vi "set active buffer.vi"(8 "error in (no error)":errorcluster, 11 "Thorcam in":refnum<class "Thorcam.lvclass">) -> (0 "error out":errorcluster, 3 "Thorcam out":refnum<class "Thorcam.lvclass">)   [LabVIEW 2012, in "Thorcam.lvclass"]
uses:
  Thorcam.lvclass
  Thorcam.lvclass/Thorcam.ctl
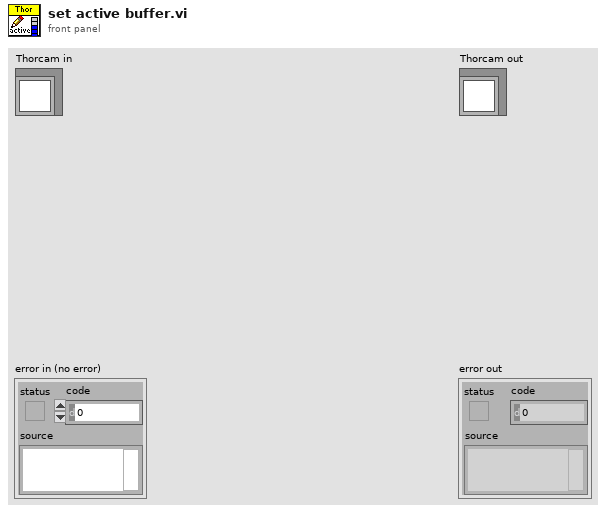
[diagram p1: front panel]
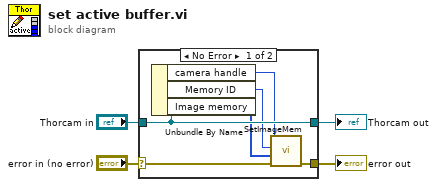
[diagram p0: block diagram]
diagram:
  n1 = case shown="No Error" "error in (no error)" {
    selector: "error in (no error)" -> [w8 w12]
    tunnel: [w7 w12] -> w3
    tunnel: [w10 w11] -> w1
    tunnel: "Thorcam in" -> [w10 w11]
    frame No Error {
      n2 = Unbundle By Name(w10) -> ("camera handle"=w9:u32, "Memory ID"=w6:i32, "Image memory"=w5:u8[])
      n3 = call <instrlib>:"SetImageMem.vi"("error in"=w8, "Image Memory In"=w5, "Memory ID In"=w6, "Camera Handle In"=w9) -> ("error out"=w7:errorcluster)  [unwired: 4 in, 3 out]
    }
    frame Error {
    }
  }
  "error out" <- w3
  "Thorcam out" <- w1
